vi "Drive PID 2014.vi"(0 "Drive":T3, 1 "Speed Limits":T24={"Turn Speed Limits"={"upper limit"=1.0, "lower limit"=1.0}, "Straight Speed Limits"={"upper limit"=1.0, "lower limit"=1.0}}, 3 "Turn Only?":bool, 5 "Setpoints":T26, 9 "From Shift":T1, 11 "error in (no error)":errorcluster, 12 "PID Gains":T25, 13 "reinitialize? (F)":bool, 14 "Deadbands":T2) -> (4 "Drive out":T3, 6 "In Range in time":bool, 8 "Commanded speeds":cluster{"Steer":dbl, "Throttle":dbl}, 10 "To Shift":T1, 15 "error out":errorcluster)   [LabVIEW 2013]
uses:
  Drive Code/Drive typedef.ctl
  Drive Code/Drive Motors Typedef.ctl
  Drive Code/GearBox Typedef.ctl
  <vilib>/Rock Robotics/WPI/MotorControl/WPI_MotorControlDeviceRef.ctl
  <vilib>/Rock Robotics/SystemInterfaces/Typedef/FPGA_TypedefDigitalModule.ctl
  <vilib>/Rock Robotics/SystemInterfaces/DIO/FPGA_DIOPWMChannel.ctl
  <vilib>/Rock Robotics/WPI/PWM/WPI_PWMDeadband.ctl
  <vilib>/Rock Robotics/WPI/CAN/Jaguar/SubVIs/WPI_CANJaguar_ControlMode.ctl
  <vilib>/Rock Robotics/WPI/PWM/WPI_PWMTransform_ConPane.ctl
  <vilib>/Rock Robotics/WPI/Solenoid/WPI_SolenoidDevRef.ctl
  <vilib>/Rock Robotics/SystemInterfaces/Typedef/FPGA_TypedefSolenoidModule.ctl
  <vilib>/Rock Robotics/WPI/Solenoid/WPI_SolenoidChannel.ctl
  Drive Code/Drive Sensor Typedef.ctl
  <vilib>/Rock Robotics/WPI/Encoder/WPI_EncoderDevRef.ctl
  <vilib>/Rock Robotics/SystemInterfaces/Encoder/FPGA_EncoderIdx.ctl
  <vilib>/Rock Robotics/SystemInterfaces/Counter/FPGA_CounterCtrSystemIndex.ctl
  <vilib>/Rock Robotics/WPI/Encoder/WPI_EncoderType.ctl
  <vilib>/Rock Robotics/WPI/Gyro/WPI_GyroDevRef.ctl
  <vilib>/Rock Robotics/SystemInterfaces/Typedef/FPGA_TypedefAnalogModule.ctl
  <vilib>/Rock Robotics/SystemInterfaces/AI/FPGA_AIChannel.ctl
  <vilib>/Rock Robotics/WPI/Solenoid/WPI_SolenoidValue.ctl
  <vilib>/Rock Robotics/WPI/Solenoid/WPI_SolenoidGetEnum.vi
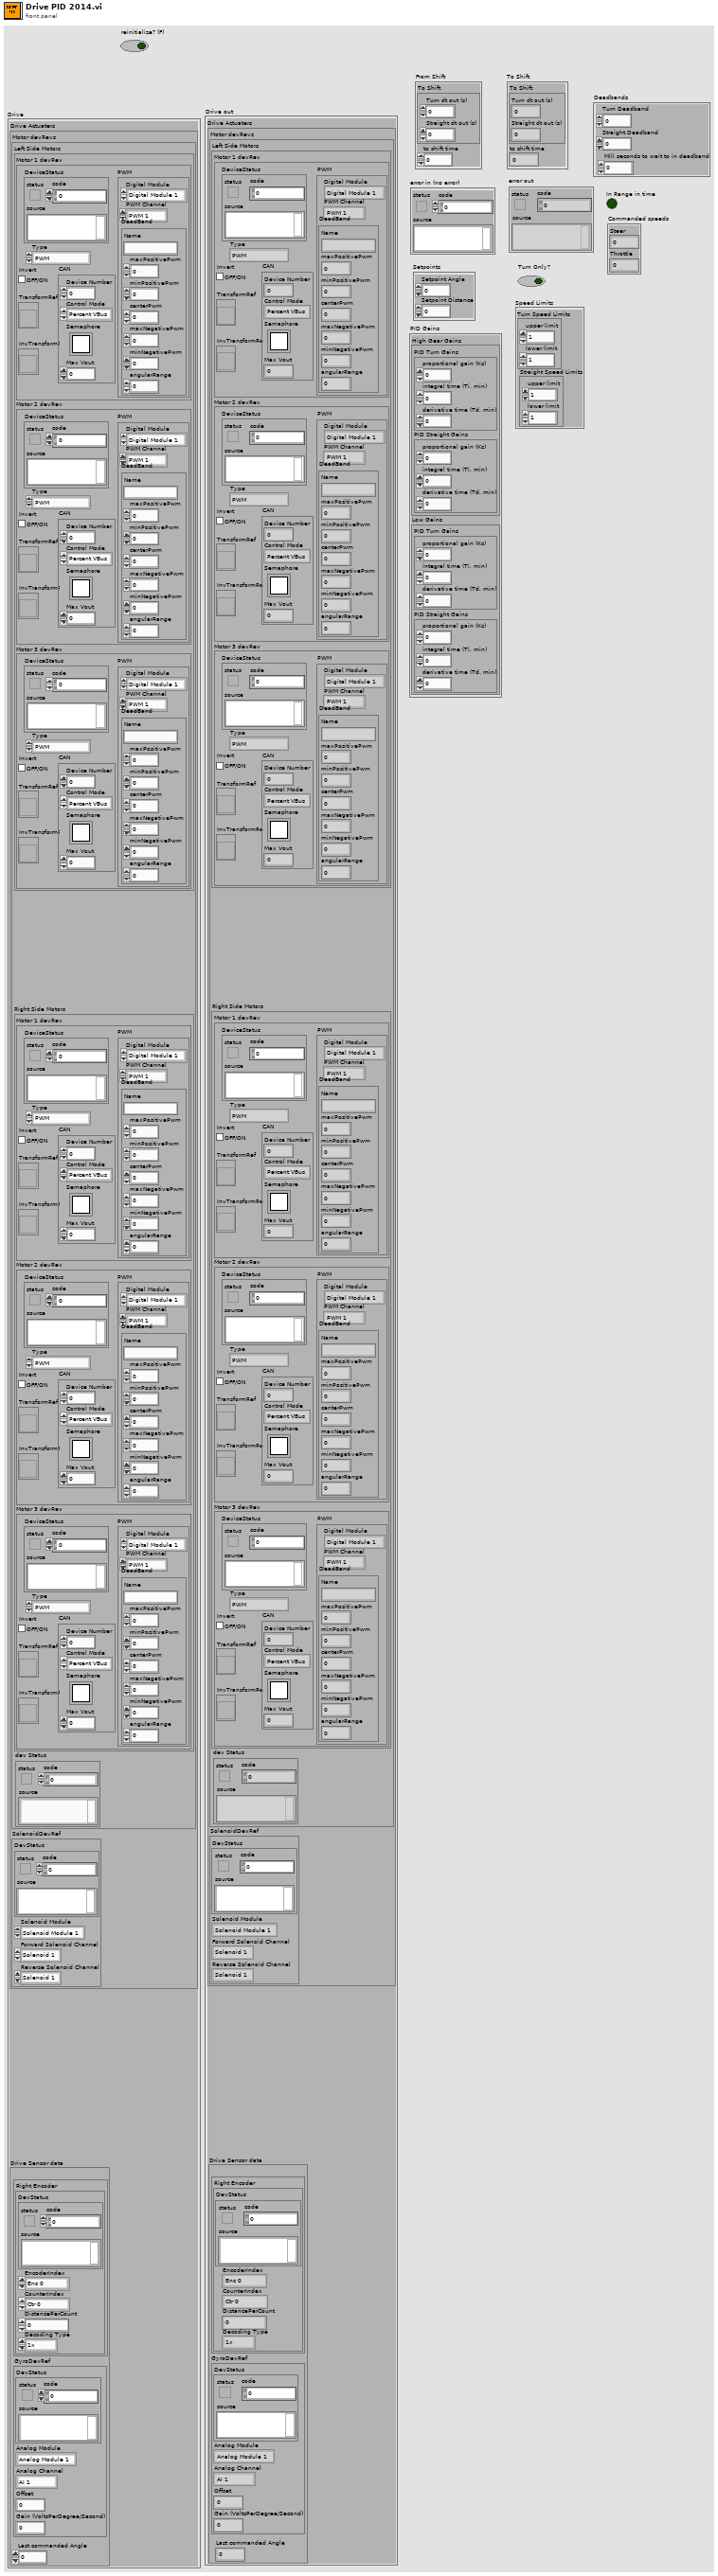
[diagram p1: front panel]
types:
  T1 = cluster{"To Shift":cluster{"Turn dt out (s)":dbl, "Straight dt out (s)":dbl}, "to shift time":u32}
  T2 = cluster{"Turn Deadband":dbl, "Straight Deadband":dbl, "Mili seconds to wait to in deadband":u32}
  T3 = typedef "Drive typedef.ctl" = cluster{"Drive Actuaters":cluster{"Motor devRevs":T4, "SolenoidDevRef":T13}, "Drive Sensor data":T16}
  T4 = typedef "Drive Motors Typedef.ctl" = cluster{"Left Side Motors":T5, "Right Side Motors":T5, "dev Status":errorcluster}
  T5 = typedef "GearBox Typedef.ctl" = cluster{"Motor 1 devRev":T6, "Motor 2 devRev":T6, "Motor 3 devRev":T6}
  T6 = typedef "WPI_MotorControlDeviceRef.ctl" = cluster{"DeviceStatus":errorcluster, "Type":enum16{"PWM", "CAN"}, "PWM":cluster{"Digital Module":T7, "PWM Channel":T8, "DeadBand":T9}, "CAN":cluster{"Device Number":u8, "Control Mode":T10, "Semaphore":T11, "Max Vout":dbl}, "Invert":bool, "TransformRef":T12, "InvTransformRef":T12}
  T7 = typedef "FPGA_TypedefDigitalModule.ctl" = enum16{"Digital Module 1", "Digital Module 2"}
  T8 = typedef "FPGA_DIOPWMChannel.ctl" = enum8{"PWM 1", "PWM 2", "PWM 3", "PWM 4", "PWM 5", "PWM 6", "PWM 7", "PWM 8", "PWM 9", "PWM 10", "Invalid"}
  T9 = typedef "WPI_PWMDeadband.ctl" = cluster{"Name":string, "maxPositivePwm":i32, "minPositivePwm":i32, "centerPwm":i32, "maxNegativePwm":i32, "minNegativePwm":i32, "angularRange":u16}
  T10 = typedef "WPI_CANJaguar_ControlMode.ctl" = enum8{"Percent VBus", "Current", "Speed", "Position", "Voltage"}
  T11 = typedef "Semaphore RefNum" = refnum<k1>
  T12 = typedef "WPI_PWMTransform_ConPane.ctl" = refnum<vi>
  T13 = typedef "WPI_SolenoidDevRef.ctl" = cluster{"DevStatus":errorcluster, "Solenoid Module":T14, "Forward Solenoid Channel":T15, "Reverse Solenoid Channel":T15}
  T14 = typedef "FPGA_TypedefSolenoidModule.ctl" = enum16{"Solenoid Module 1", "Solenoid Module 2"}
  T15 = typedef "WPI_SolenoidChannel.ctl" = enum8{"Solenoid 1", "Solenoid 2", "Solenoid 3", "Solenoid 4", "Solenoid 5", "Solenoid 6", "Solenoid 7", "Solenoid 8", "Invalid"}
  T16 = typedef "Drive Sensor Typedef.ctl" = cluster{"Encoders":cluster{"Right Encoder":T17}, "GyroDevRef":T21, "Last commanded Angle":dbl}
  T17 = typedef "WPI_EncoderDevRef.ctl" = cluster{"DevStatus":errorcluster, "EncoderIndex":T18, "CounterIndex":T19, "DistancePerCount":dbl, "Decoding Type":T20}
  T18 = typedef "FPGA_EncoderIdx.ctl" = enum8{"Enc 0", "Enc 1", "Enc 2", "Enc 3", "Invalid"}
  T19 = typedef "FPGA_CounterCtrSystemIndex.ctl" = enum8{"Ctr 0", "Ctr 1", "Ctr 2", "Ctr 3", "Ctr 4", "Ctr 5", "Ctr 6", "Ctr 7", "Invalid"}
  T20 = typedef "WPI_EncoderType.ctl" = enum16{"1x", "2x", "4x"}
  T21 = typedef "WPI_GyroDevRef.ctl" = cluster{"DevStatus":errorcluster, "Analog Module":T22, "Analog Channel":T23, "Offset":dbl, "Gain (VoltsPerDegree/Second)":dbl}
  T22 = typedef "FPGA_TypedefAnalogModule.ctl" = enum16{"Analog Module 1", "Analog Module 2"}
  T23 = typedef "FPGA_AIChannel.ctl" = enum8{"AI 1", "AI 2", "AI 3", "AI 4", "AI 5", "AI 6", "AI 7", "AI 8", "Invalid"}
  T24 = cluster{"Turn Speed Limits":cluster{"upper limit":dbl, "lower limit":dbl}, "Straight Speed Limits":cluster{"upper limit":dbl, "lower limit":dbl}}
  T25 = cluster{"High Gear Gains":cluster{"PID Turn Gains":cluster{"proportional gain (Kc)":dbl, "integral time (Ti, min)":dbl, "derivative time (Td, min)":dbl}, "PID Straight Gains":cluster{"proportional gain (Kc)":dbl, "integral time (Ti, min)":dbl, "derivative time (Td, min)":dbl}}, "Low Gains":cluster{"PID Turn Gains":cluster{"proportional gain (Kc)":dbl, "integral time (Ti, min)":dbl, "derivative time (Td, min)":dbl}, "PID Straight Gains":cluster{"proportional gain (Kc)":dbl, "integral time (Ti, min)":dbl, "derivative time (Td, min)":dbl}}}
  T26 = cluster{"Setpoint Angle":dbl, "Setpoint Distance":dbl}
  T27 = typedef "WPI_SolenoidValue.ctl" = enum16{"Off", "On", "Forward", "Reverse"}
  T28 = cluster{"Motor devRevs":T4, "SolenoidDevRef":T13}
  T29 = cluster{"Turn dt out (s)":dbl, "Straight dt out (s)":dbl}
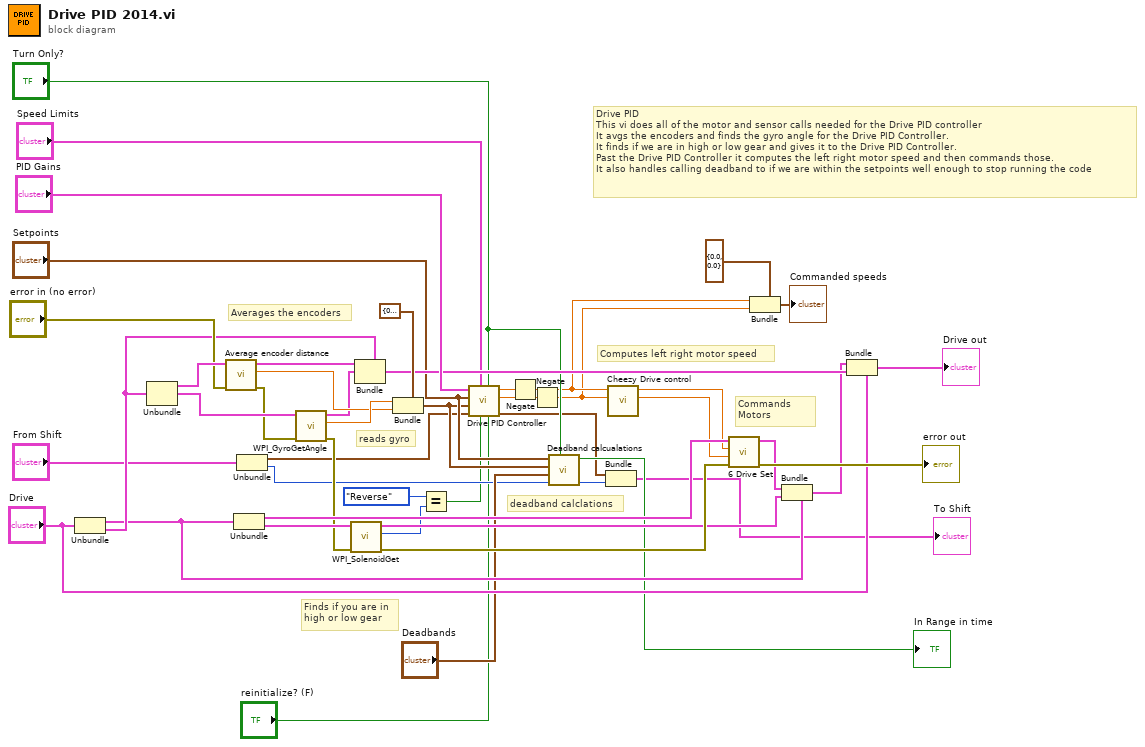
[diagram p0: block diagram]
diagram:
  # "reads gyro"
  # "Averages the encoders"
  # "Finds if you are in\nhigh or low gear"
  # "deadband calclations"
  # "Commands Motors"
  # "Computes left right motor speed"
  # "Drive PID\nThis vi does all of the motor and sensor calls needed for the Drive PID controller\nIt avgs the encoders and finds the gyro angle for the Drive PID Controller.\nIt finds if we are in high or low gear and gives it to the Drive PID Controller.\nPast the Drive PID Controller it computes the left right motor speed and then commands those.\nIt also handles calling deadband to if we are within the setpoints well enough to stop running the code"
  n1 = Unbundle("Drive") -> ("Drive Actuaters"=w27:T28, "Drive Sensor data"=w32:T16)
  n2 = Unbundle(w32) -> ("Encoders"=w44:cluster{"Right Encoder":T17}, "GyroDevRef"=w42:T21)  [unwired: 1 out]
  n3 = call "Average encoder distance.vi"("error in (no error)"="error in (no error)", "Encoders"=w44) -> ("error out"=w38:errorcluster, "Average encoder distance"=w39:dbl, "Encoders"=w31:cluster{"EncoderDevRef":T17})  [unwired: 7 in]
  n4 = Unbundle(w27) -> ("Motor devRevs"=w47:T4, "SolenoidDevRef"=w43:T13)
  n5 = Unbundle("From Shift") -> ("To Shift"=w12:T29, "to shift time"=w11:u32)
  n6 = call <vilib>:"WPI_GyroGetAngle.vi"("error in (no error)"=w38, "GyroDevRef"=w42) -> ("error out"=w37:errorcluster, "Angle"=w40:dbl, "GyroDevRef"=w30:T21)  [unwired: 6 in, 1 out]
  n7 = call-poly <vilib>:"WPI_SolenoidGet.vi"("error in (no error)"=w37, "SolenoidDevRef"=w43) -> ("error out"=w36:errorcluster, "Value"=w6:T27, "SolenoidDevRef"=w23:T13)  [unwired: 7 in]
  n8 = Bundle(cluster=w32, "Encoders"=w31, "GyroDevRef"=w30) -> (w28:T16)  [unwired: 1 in]
  n9 = Bundle(cluster=cluster{"Angle":dbl, "Encoder Distance":dbl} {"Angle"=0.0, "Encoder Distance"=0.0} ("Procces Variable"), "Angle"=w40, "Encoder Distance"=w39) -> (w20:cluster{"Angle":dbl, "Encoder Distance":dbl})
  n10 = Equal?(x=WPI_SolenoidValue."Reverse", y=w6) -> (x = y?=w4:bool)
  n11 = call "Drive PID Controller.vi"("reinitialize? (F)"="reinitialize? (F)", "Turn Only?"="Turn Only?", "High Gear?"=w4, "Speed Limits"="Speed Limits", "From Shift"=w12, "Procces Variable"=w20, "Setpoints"="Setpoints", "PID Gains"="PID Gains") -> ("To Shift"=w16:T29, "Throttle output"=w8:dbl, "Steer ouput"=w9:dbl)  [unwired: 1 in]
  n12 = Negate(x=w9) -> (-x=w3:dbl)
  n13 = Negate(x=w8) -> (-x=w2:dbl)
  n14 = call "Deadband calcualations.vi"("Turn Only"="Turn Only?", "From shift time"=w11, "Deadbands"="Deadbands", "Procces Variables"=w20, "Setpoints"="Setpoints") -> ("to shift time"=w15:u32, "In Range in time"=→"In Range in time":bool)  [unwired: 4 in, 1 out]
  n15 = Bundle("To Shift"=w16, "to shift time"=w15) -> (→"To Shift":T1)  [unwired: 1 in]
  n16 = call "Cheezy Drive control.vi"("Throttle"=w2, "Steer"=w3) -> ("Right motor output"=w45:dbl, "Left motor ouput"=w46:dbl)  [unwired: 8 in]
  n17 = call "6 Drive Set.vi"("Motor devRevs"=w47, "Left side speed"=w46, "Right side speed"=w45, "error in (no error)"=w36) -> ("Motor devRevs"=w26:T4, "error out"=→"error out":errorcluster)  [unwired: 5 in]
  n18 = Bundle(cluster=cluster{"Steer":dbl, "Throttle":dbl} {"Steer"=0.0, "Throttle"=0.0} ("Commanded speeds"), "Steer"=w3, "Throttle"=w2) -> (→"Commanded speeds":cluster{"Steer":dbl, "Throttle":dbl})
  n19 = Bundle(cluster=w27, "Motor devRevs"=w26, "SolenoidDevRef"=w23) -> (w24:T28)
  n20 = Bundle(cluster="Drive", "Drive Actuaters"=w24, "Drive Sensor data"=w28) -> (→"Drive out":T3)
